vi "Convert CTRE Encoder Velocity to RPM.vi"(10 "Units/ Rev":dbl, 11 "CTRE Vel (units/.1S)":dbl) -> (3 "RPM Out":dbl)   [LabVIEW 2023, in "RingPlacer_ACT.lvlib"]
uses:
  RingPlacer_ACT.lvlib
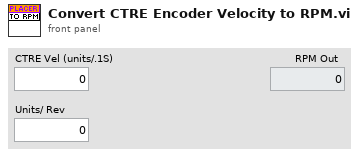
[diagram p1: front panel]
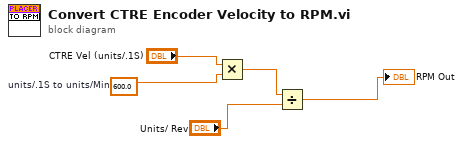
[diagram p0: block diagram]
diagram:
  w5 = 600.0  # units/.1S to units/Min
  n1 = Multiply(x="CTRE Vel (units/.1S)", y=w5) -> (x*y=w3:dbl)
  n2 = Divide(x=w3, y="Units/ Rev") -> (x/y=→"RPM Out":dbl)
